vi "Sort.vi"(2 "Amplitudes":dbl[](array[numeric])=[-93.89816560613959], 3 "Locations":dbl[](array[numeric])=[115.85354561961238]) -> (0 "amplitude":dbl=-93.89816560613959, 1 "location":dbl=115.85354561961238)   [LabVIEW 2018]
panel:
  in  "bypass":bool
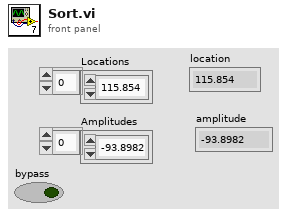
[diagram p1: front panel]
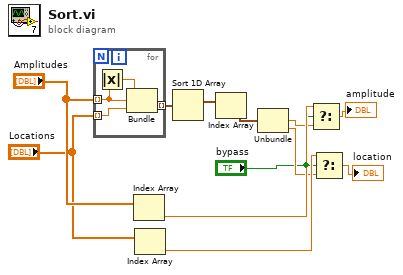
[diagram p0: block diagram]
diagram:
  n1 = for {
    tunnel: "Amplitudes" -> [w13] mode=indexing
    tunnel: "Locations" -> [w15] mode=indexing
    tunnel: [w16] -> w11 mode=indexing
    n2 = Absolute Value(x=w13) -> (abs(x)=w14:dbl)
    n3 = Bundle(w14, w13, w15) -> (w16:cluster{dbl, dbl, dbl})  [unwired: 1 in]
  }
  n4 = Index Array(array="Amplitudes") -> (element=w6:dbl)  [unwired: 1 in]
  n5 = Index Array(array="Locations") -> (element=w3:dbl)  [unwired: 1 in]
  n6 = Sort 1D Array(array=w11) -> (sorted array=w12:cluster{dbl, dbl, dbl}[])
  n7 = Index Array(array=w12) -> (element=w10:cluster{dbl, dbl, dbl})  [unwired: 1 in]
  n8 = Unbundle(w10) -> (w5:dbl, w2:dbl)  [unwired: 1 out]
  n9 = Select(t=w6, s="bypass", f=w5) -> (s? t:f=→"amplitude":dbl)
  n10 = Select(t=w3, s="bypass", f=w2) -> (s? t:f=→"location":dbl)
